vi "get device count.vi"(8 "error in (no error)":errorcluster, 11 "device_enumeration":u32) -> (0 "error out":errorcluster, 3 "function return":i32)   [LabVIEW 2012, in "libximc.lvlib"]
doc: "int XIMC_API get_device_count(device_enumeration_t device_enumeration);"
uses:
  libximc.lvlib
  libximc.dll
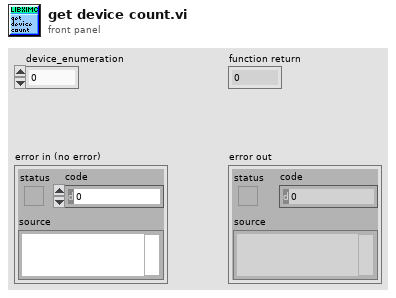
[diagram p1: front panel]
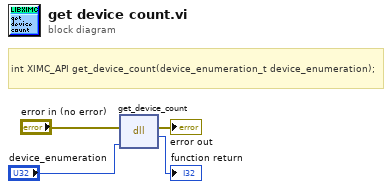
[diagram p0: block diagram]
diagram:
  # "int XIMC_API get_device_count(device_enumeration_t device_enumeration);"
  n1 = dll-call lib="C:/Users/user/Desktop/labview-2.9.11-gen/libximc.*" fn="get_device_count"(error in="error in (no error)", "device_enumeration"="device_enumeration") -> (error out=→"error out":errorcluster, →"function return":i32)  [unwired: 3 in, 1 out]
